vi "Set Color.vi"(8 "error in (no error)":errorcluster, 10 "Color Message.lvclass":refnum<class "Color Message.lvclass">, 11 "Color Interface in":refnum<class "Color Interface.lvclass">) -> (0 "error out":errorcluster, 3 "Color Interface out":refnum<class "Color Interface.lvclass">)   [LabVIEW 2020, in "Color Interface.lvclass"]
uses:
  Color Interface.lvclass
  Color/Color Message.lvclass
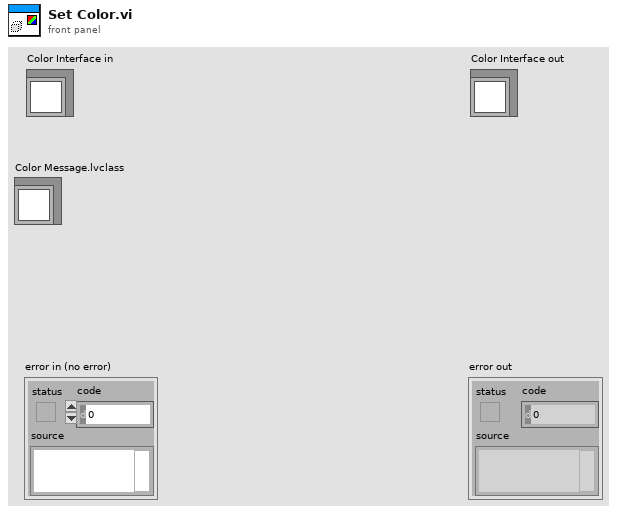
[diagram p1: front panel]
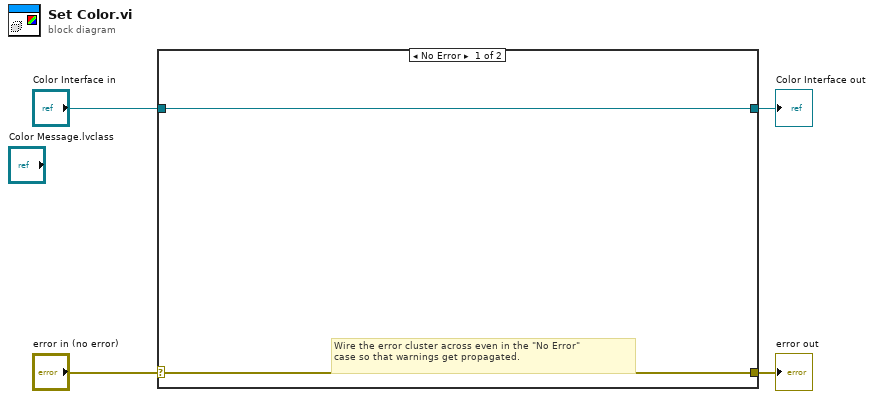
[diagram p0: block diagram]
diagram:
  n1 = case shown="No Error" "error in (no error)" {
    selector: "error in (no error)" -> [w5 w8]
    tunnel: [w5 w8] -> w3
    tunnel: [w6 w7] -> w1
    tunnel: "Color Interface in" -> [w6 w7]
    frame No Error {
      # "Wire the error cluster across even in the \"No Error\"\ncase so that warnings get propagated."
    }
    frame Error {
    }
  }
  "error out" <- w3
  "Color Interface out" <- w1
